vi "DUT On Logic.vi"(0 "Boolean in":refnum<vi>, 1 "reference in":refnum<vi>, 2 "Mfg. Date:":timestamp=timestamp(3431055600 s since 1904-01-01) format="%<%m/%d/%Y>T", 7 "reference 3":refnum<vi>, 9 "DeviceParameters":T1 {"DevInfo"."ASICtrim" format="%02x"}, 12 "reference 4":refnum<vi>, 13 "State-machine Local Variables in":T3={"Message"="", "Homed?"=FALSE, "NextState"=enum."Timeout", "G.Load"=1.0, "G.Position"=0.0, "Load#"=0, "[G.Loads]"=[], "[TotalLoads]"=[], "[Errors]"=[], "ZeroWait"=0, "Results"=[], "DwellWait"=FALSE, "Test Result"=FALSE, "[CondyleLoads]"=[], "[Max]"=[], "[Min]"=[], "Valid String?"=FALSE, "ScanTime"=timestamp(0 s since 1904-01-01), "ScannedString"="", "LabelDevID"=0, "MfgDate"=timestamp(0 s since 1904-01-01), "[EEPROM Cmds]"=[], "[CalData]"=[], "[A/Ds]"=[], "[A/Dmax]"=[], "[A/Dmin]"=[], "BattMax"=0.0, "BattMin"=0.0, "DwellTime"=0, "PendingDeviceType"="", "Zero G.load"=0.0, "GAINC Value"="", "Programming Step"=enum."Load EEPROM", "Front Panel Program?"=FALSE, "Final Program?"=FALSE, "PCB Score"=100, "AssyScore"=100, "Pass/Fail #"="", "Result String"="", "Programming Mode"=enum."Initial Program", "Angle Test Step"=enum."Get Y", "Accel Values"=[], "Shutdown Counter"=0, "V1"=0, "V2"=5, "V3"=0, "V4"=0, "EEPROM Data"=[], "Counter"=0, "Page#"=0, "Timer"=timestamp(0 s since 1904-01-01), "Use Mark10?"=FALSE, "Eng-Result#"=0, "DUT Serial #"=0, "Scroll Message?"=FALSE, "Clear Message"=FALSE, "Batt Test Step "=enum."Initialize", "RXTX Window Found?"=FALSE, "Shutdown First Call?"=FALSE, "A2 Delay (msec)"=0, "Support Script"={"Script #"="", "Script Revision"="", "[OEMs]"=[], "[[DeviceTypes]]"=[], "[[DeviceTypesVals]]"=[], "[[List of Errors]]"=[], "Default GAINC"="", "[[ASICtrims]]"=[], "ID For Echo"="", "Condyle A CalFactor"=100, "Condyle B CalFactor"=100, "[OEMs Prefix]"=[], "Packet ID 18"="", "[[Force Table Load Test]]"=[], "[[Force Table AccurTest]]"=[]}, "Serial Table"={"Serial File Path"=path "", "[[Serial Lookup Table]]"=[], "Serial Device Info"=[], "Valid Serial?"=FALSE}, "Target Information"={"Target Brand"="", "Target DeviceType"="", "Target Serial#"=100, "Target Lot#"=0, "Target DevID"=0, "Target Channel"=5}, "Operator"="", "COM Port"="", "Config Path"=path "", "Tx Array"=[], "DUT Parameters"={"Channel"=0, "DeviceID"=0, "Script Rev"=0, "Month"=0, "Day"=0, "Year"=0, "Lot#"=0, "V1"=0, "V2"=0, "V3"=0, "V4"=0, "MFG"=0, "Cal FactorA"=0, "Cal FactorB"=0, "ASICtrim"=[], "TmpChan"=0, "GAINC"="", "Brand"="", "Device"="", "Serial #"=0, "Batt310"=0, "Batt 280"=0}, "FTS Main?"=FALSE, "Loading"={"[Forces]"=[], "[Dwell]"=[], "Loading Step"=enum."Initialize Test"}, "Software Version"="", "Correction Factor"="", "Second Load Test"=FALSE, "Acc Loads"=[], "Mark10 Config"={"H2S%"=[80.0, 85.0, 90.0, 95.0, 100.0], "H2S Speed"=[12.0, 8.0, 6.0, 4.0, 2.0], "H to S"=2.0, "Home Speed"=1.0, "LoadWin"=0.0, "Load Speed"=0.0, "PID"={"Kp"=0.04, "Kd"=0.005001, "Ki"=2.9999999999999923e-05}}, "Channels"={"Transceiver Ch"=5, "Operating Ch"=5, "Start Ch"=0}} {"Mark10 Config"."PID"."Ki" min=0.0 max=200.0 format="%.6f"; "Mark10 Config"."PID"."Kd" min=0.0 max=200.0 format="%.6f"; "Mark10 Config"."PID"."Kp" min=0.0 max=200.0 format="%.6f"; "DUT Parameters"."ASICtrim" format="%02x"}, 14 "New Data":bool) -> (4 "Main Data out":T3={"Message"="", "Homed?"=FALSE, "NextState"=enum."Timeout", "G.Load"=1.0, "G.Position"=0.0, "Load#"=0, "[G.Loads]"=[], "[TotalLoads]"=[], "[Errors]"=[], "ZeroWait"=0, "Results"=[], "DwellWait"=FALSE, "Test Result"=FALSE, "[CondyleLoads]"=[], "[Max]"=[], "[Min]"=[], "Valid String?"=FALSE, "ScanTime"=timestamp(0 s since 1904-01-01), "ScannedString"="", "LabelDevID"=0, "MfgDate"=timestamp(0 s since 1904-01-01), "[EEPROM Cmds]"=[], "[CalData]"=[], "[A/Ds]"=[], "[A/Dmax]"=[], "[A/Dmin]"=[], "BattMax"=0.0, "BattMin"=0.0, "DwellTime"=0, "PendingDeviceType"="", "Zero G.load"=0.0, "GAINC Value"="", "Programming Step"=enum."Load EEPROM", "Front Panel Program?"=FALSE, "Final Program?"=FALSE, "PCB Score"=100, "AssyScore"=100, "Pass/Fail #"="", "Result String"="", "Programming Mode"=enum."Initial Program", "Angle Test Step"=enum."Get Y", "Accel Values"=[], "Shutdown Counter"=0, "V1"=0, "V2"=5, "V3"=0, "V4"=0, "EEPROM Data"=[], "Counter"=0, "Page#"=0, "Timer"=timestamp(0 s since 1904-01-01), "Use Mark10?"=FALSE, "Eng-Result#"=0, "DUT Serial #"=0, "Scroll Message?"=FALSE, "Clear Message"=FALSE, "Batt Test Step "=enum."Initialize", "RXTX Window Found?"=FALSE, "Shutdown First Call?"=FALSE, "A2 Delay (msec)"=0, "Support Script"={"Script #"="", "Script Revision"="", "[OEMs]"=[], "[[DeviceTypes]]"=[], "[[DeviceTypesVals]]"=[], "[[List of Errors]]"=[], "Default GAINC"="", "[[ASICtrims]]"=[], "ID For Echo"="", "Condyle A CalFactor"=100, "Condyle B CalFactor"=100, "[OEMs Prefix]"=[], "Packet ID 18"="", "[[Force Table Load Test]]"=[], "[[Force Table AccurTest]]"=[]}, "Serial Table"={"Serial File Path"=path "", "[[Serial Lookup Table]]"=[], "Serial Device Info"=[], "Valid Serial?"=FALSE}, "Target Information"={"Target Brand"="", "Target DeviceType"="", "Target Serial#"=100, "Target Lot#"=0, "Target DevID"=0, "Target Channel"=5}, "Operator"="", "COM Port"="", "Config Path"=path "", "Tx Array"=[], "DUT Parameters"={"Channel"=0, "DeviceID"=0, "Script Rev"=0, "Month"=0, "Day"=0, "Year"=0, "Lot#"=0, "V1"=0, "V2"=0, "V3"=0, "V4"=0, "MFG"=0, "Cal FactorA"=0, "Cal FactorB"=0, "ASICtrim"=[], "TmpChan"=0, "GAINC"="", "Brand"="", "Device"="", "Serial #"=0, "Batt310"=0, "Batt 280"=0}, "FTS Main?"=FALSE, "Loading"={"[Forces]"=[], "[Dwell]"=[], "Loading Step"=enum."Initialize Test"}, "Software Version"="", "Correction Factor"="", "Second Load Test"=FALSE, "Acc Loads"=[], "Mark10 Config"={"H2S%"=[80.0, 85.0, 90.0, 95.0, 100.0], "H2S Speed"=[12.0, 8.0, 6.0, 4.0, 2.0], "H to S"=2.0, "Home Speed"=1.0, "LoadWin"=0.0, "Load Speed"=0.0, "PID"={"Kp"=0.04, "Kd"=0.005001, "Ki"=2.9999999999999923e-05}}, "Channels"={"Transceiver Ch"=5, "Operating Ch"=5, "Start Ch"=0}} {"Mark10 Config"."PID"."Ki" min=0.0 max=200.0 format="%.6f"; "Mark10 Config"."PID"."Kd" min=0.0 max=200.0 format="%.6f"; "Mark10 Config"."PID"."Kp" min=0.0 max=200.0 format="%.6f"; "DUT Parameters"."ASICtrim" format="%02x"})   [LabVIEW 2013]
uses:
  Controls/Gen2 FT Globals.vi
  Controls/Gen2 FT states.ctl
  Controls/Iniial Device Programming.ctl
  ProgramStageControl.ctl
  Controls/LocalVars.ctl
  Controls/InfoPacket.ctl
  Controls/DeviceInfo.ctl
  Controls/Batt Cap Steps.ctl
  Controls/Support Script.ctl
  Controls/Serial Table.ctl
  Controls/Device Information.ctl
  Controls/Load Step.ctl
  Controls/Loading.ctl
  Controls/PID parameters.ctl
  Controls/Mark10 Config.ctl
  Controls/Channels.ctl
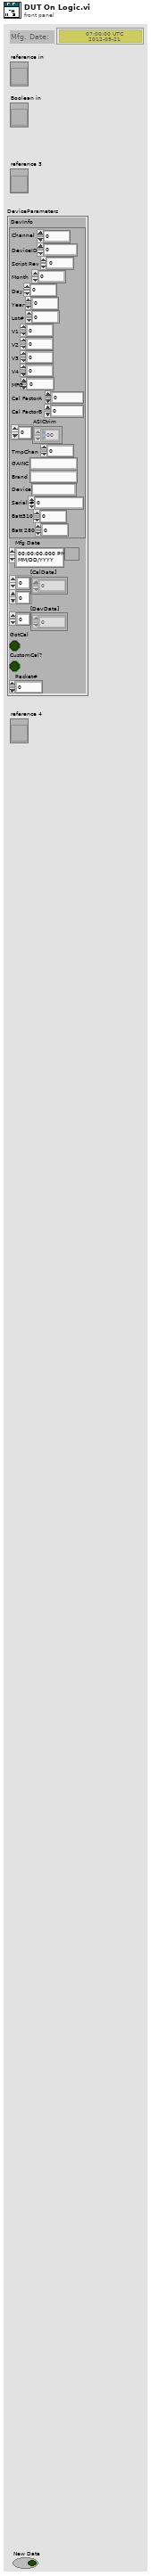
[diagram p1: front panel]
types:
  T1 = typedef "DeviceInfo.ctl" = cluster{"DevInfo":T2, "Mfg Date":timestamp, "[CalData]":u8[][], "[DevData]":u8[], "GotCal":bool, "CustomCal?":bool, "Packet#":i32}
  T2 = typedef "InfoPacket.ctl" = cluster{"Channel":u8, "DeviceID":u32, "Script Rev":u8, "Month":u8, "Day":u8, "Year":u8, "Lot#":u32, "V1":u16, "V2":u16, "V3":u16, "V4":u16, "MFG":u8, "Cal FactorA":u8, "Cal FactorB":u8, "ASICtrim":u8[], "TmpChan":u8, "GAINC":string, "Brand":string, "Device":string, "Serial #":u64, "Batt310":u16, "Batt 280":u16}
  T3 = typedef "LocalVars.ctl" = cluster{"Message":string, "Homed?":bool, "NextState":T4, "G.Load":dbl, "G.Position":dbl, "Load#":i32, "[G.Loads]":dbl[], "[TotalLoads]":dbl[], "[Errors]":dbl[][], "ZeroWait":u32, "Results":dbl[], "DwellWait":bool, "Test Result":bool, "[CondyleLoads]":dbl[][], "[Max]":dbl[], "[Min]":dbl[], "Valid String?":bool, "ScanTime":timestamp, "ScannedString":string, "LabelDevID":u32, "MfgDate":timestamp, "[EEPROM Cmds]":u8[][], "[CalData]":u8[][], "[A/Ds]":dbl[][], "[A/Dmax]":dbl[], "[A/Dmin]":dbl[], "BattMax":dbl, "BattMin":dbl, "DwellTime":i32, "PendingDeviceType":string, "Zero G.load":dbl, "GAINC Value":string, "Programming Step":T5, "Front Panel Program?":bool, "Final Program?":bool, "PCB Score":i32, "AssyScore":i32, "Pass/Fail #":string, "Result String":string, "Programming Mode":T6, "Angle Test Step":enum16{"Initialize", "Get X", "Get Y", "Get Z", "Next Test"}, "Accel Values":dbl[][], "Shutdown Counter":u32, "V1":i32, "V2":i32, "V3":i32, "V4":i32, "EEPROM Data":i32[][], "Counter":i32, "Page#":i32, "Timer":timestamp, "Use Mark10?":bool, "Eng-Result#":u32, "DUT Serial #":i32, "Scroll Message?":bool, "Clear Message":bool, "Batt Test Step ":T7, "RXTX Window Found?":bool, "Shutdown First Call?":bool, "A2 Delay (msec)":i16, "Support Script":T8, "Serial Table":T9, "Target Information":T10, "Operator":string, "COM Port":string, "Config Path":path, "Tx Array":u8[], "DUT Parameters":T2, "FTS Main?":bool, "Loading":T11, "Software Version":string, "Correction Factor":string, "Second Load Test":bool, "Acc Loads":dbl[][], "Mark10 Config":T13, "Channels":T15}
  T4 = typedef "Gen2 FT states.ctl" = enum16{"---------SETUP-------", "Initialization", "Read Support Data", "Initialize Mark-10", "Initialize Transceiver", "------UTILITIES------", "Change DUT Channel", "Find RxTx Window", "Reset Device", "Scan Channels", "Read Serial Lookup", "Shutdown Device", "ESTOP", "--------USER---------", "Timeout", "-----PROGRAM-----", "Program Device", "------MARK10--------", "Go Home", "MoveUp", "MoveDown", "Goto Load", "Goto Position", "Stop Motor", "---------TESTS--------", "Start Test", "Angle Test", "Load Test", "Load Accuracy Test", "Battery Test", "------RESULTS-------", "End Test", "Display Result", "--------EXIT--------", "Exit"}
  T5 = typedef "Iniial Device Programming.ctl" = enum16{"Load EEPROM", "Send First A1", "Send EEPROM", "Send A1", "Check EEPROM Echo", "Verify transmission", "Programming Successful", "Programming Failed"}
  T6 = typedef "ProgramStageControl.ctl" = enum16{"Initial Program", "GainC", "Scales"}
  T7 = typedef "Batt Cap Steps.ctl" = enum16{"Initialize", "Collect 2.8 Volts", "Collect 3.1 Volts", "Check Results"}
  T8 = typedef "Support Script.ctl" = cluster{"Script #":string, "Script Revision":string, "[OEMs]":string[], "[[DeviceTypes]]":string[][], "[[DeviceTypesVals]]":u16[][], "[[List of Errors]]":string[][], "Default GAINC":string, "[[ASICtrims]]":u8[][], "ID For Echo":string, "Condyle A CalFactor":i32, "Condyle B CalFactor":i32, "[OEMs Prefix]":string[], "Packet ID 18":string, "[[Force Table Load Test]]":dbl[][], "[[Force Table AccurTest]]":dbl[][]}
  T9 = typedef "Serial Table.ctl" = cluster{"Serial File Path":path, "[[Serial Lookup Table]]":string[][], "Serial Device Info":string[], "Valid Serial?":bool}
  T10 = typedef "Device Information.ctl" = cluster{"Target Brand":string, "Target DeviceType":string, "Target Serial#":i32, "Target Lot#":u32, "Target DevID":u32, "Target Channel":u8}
  T11 = typedef "Loading.ctl" = cluster{"[Forces]":dbl[], "[Dwell]":dbl[], "Loading Step":T12}
  T12 = typedef "Load Step.ctl" = enum16{"Initialize Test", "Go Home", "Detect Dev Surface", "Wait to zero Device", "Zero Device", "Do Test", "Test Result"}
  T13 = typedef "Mark10 Config.ctl" = cluster{"H2S%":dbl[], "H2S Speed":dbl[], "H to S":dbl, "Home Speed":dbl, "LoadWin":dbl, "Load Speed":dbl, "PID":T14}
  T14 = typedef "PID parameters.ctl" = cluster{"Kp":dbl, "Kd":dbl, "Ki":dbl}
  T15 = typedef "Channels.ctl" = cluster{"Transceiver Ch":u8, "Operating Ch":u8, "Start Ch":u8}
  T16 = typedef "LVDateTimeRec.ctl" = cluster{"fractional second":dbl, "second":i32, "minute":i32, "hour":i32, "day of month":i32, "month":i32, "year":i32, "day of week":i32, "day of year":i32, "DST":i32}
  T17 = typedef "InfoPacket.ctl" = cluster{"Channel":u8, "DeviceID":u32, "Script Rev":u8, "Month":u8, "Day":u8, "Year":u8, "Lot#":u32, "V1":u16, "V2":u16, "V3":u16, "V4":u16, "MFG":u8, "Cal Factor":u8, "Cal FactorB":u8, "ASICtrim":u8[], "TmpChan":u8, "GAINC Value":string, "Brand":string, "DeviceType":string, "Serial Number":u64}
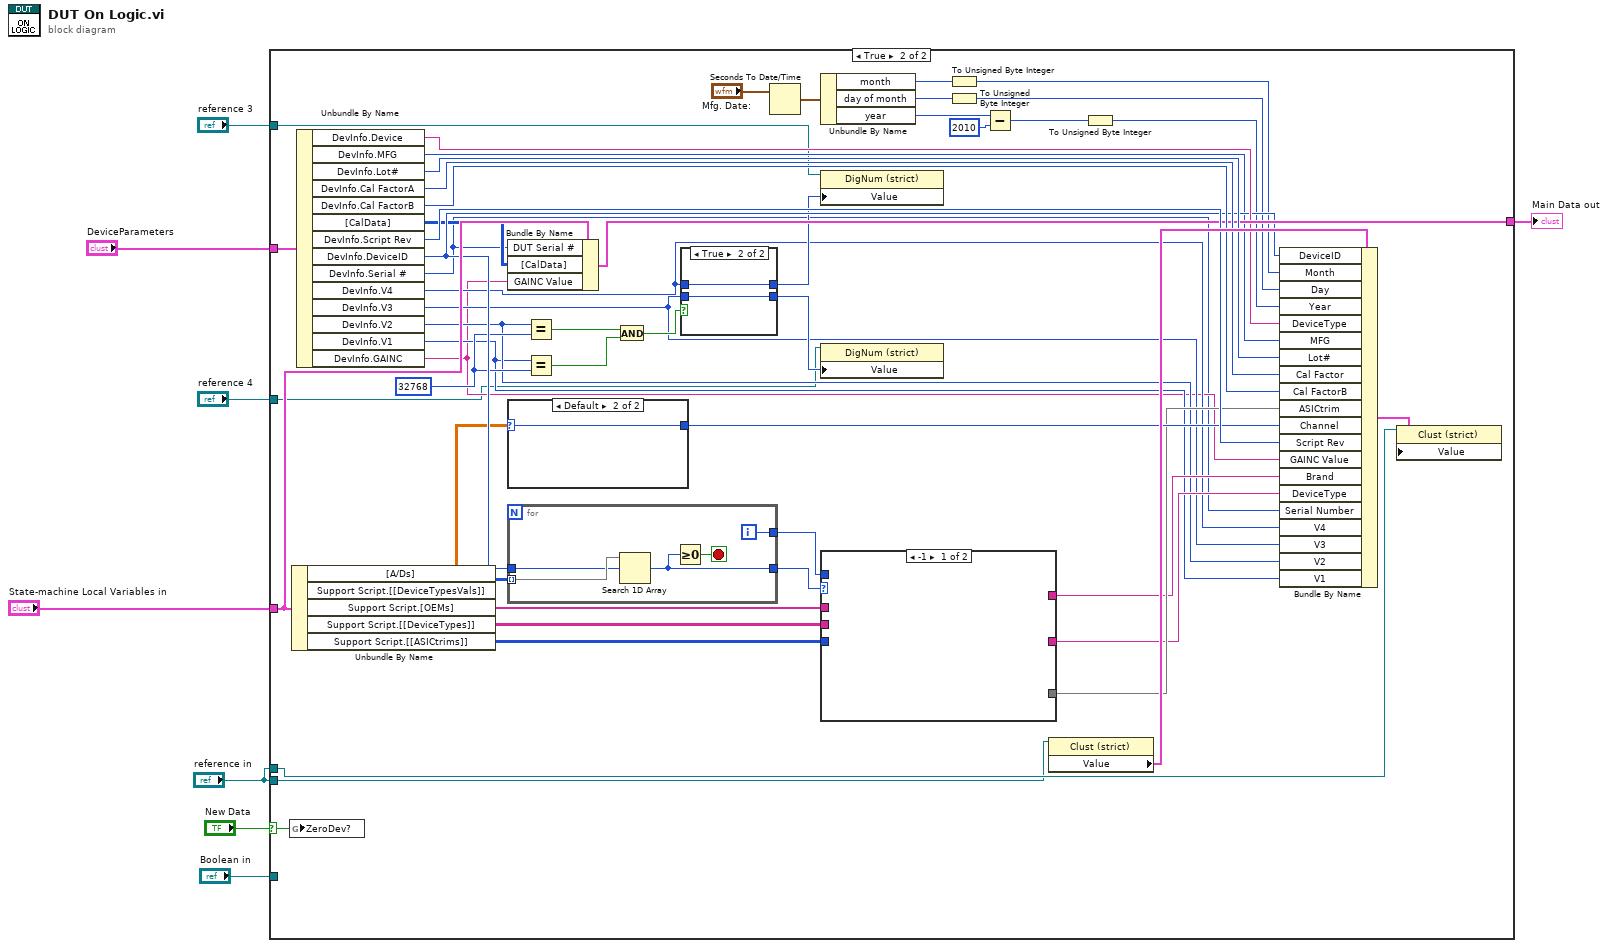
[diagram p0: block diagram]
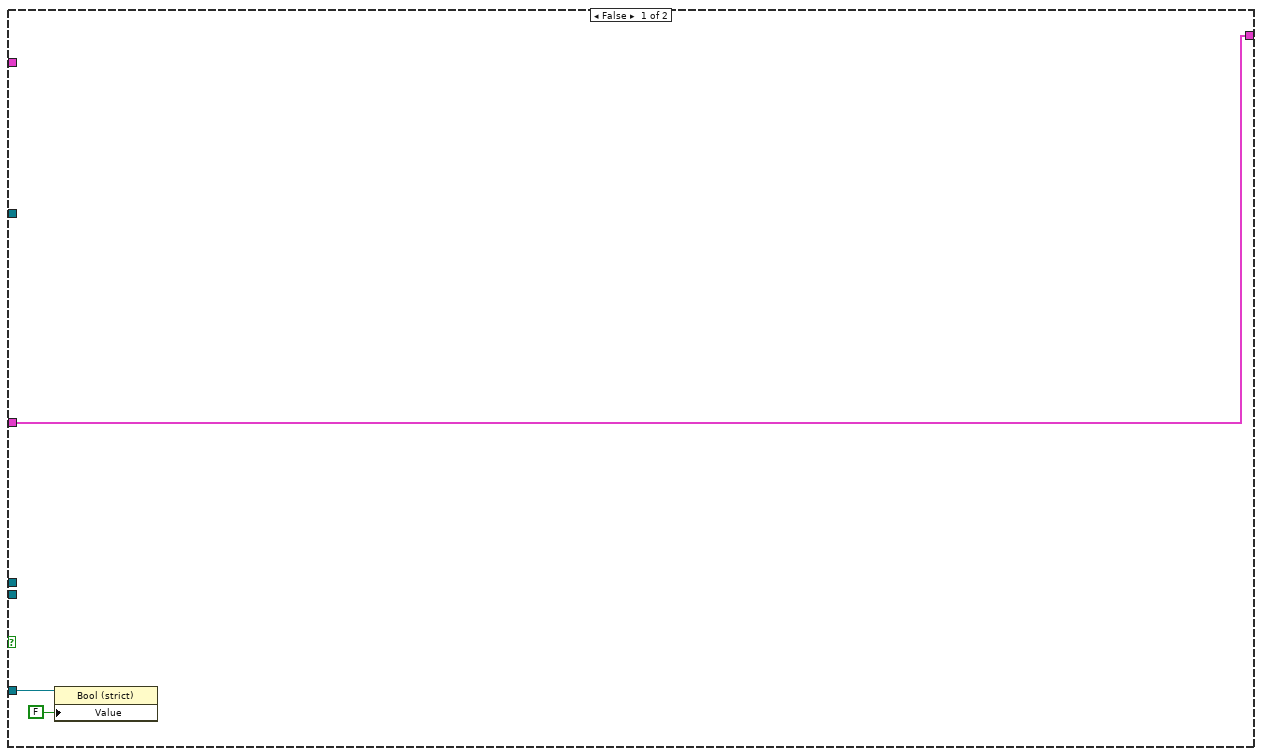
[diagram p2: hidden frame]
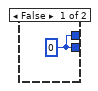
[diagram p3: hidden frame]
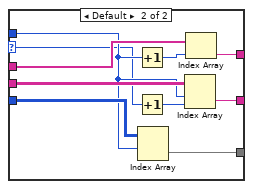
[diagram p4: hidden frame]
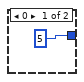
[diagram p5: hidden frame]
diagram:
  n1 = case shown="True" "New Data" {
    selector: "New Data" -> [_ w30]
    tunnel: "DeviceParameters" -> [_ w60]
    tunnel: [w11 w48] -> w6
    tunnel: "State-machine Local Variables in" -> [w11 w47]
    tunnel: "Boolean in" -> [w9 _]
    tunnel: "reference in" -> [_ w17]
    tunnel: "reference in" -> [_ w16]
    tunnel: "reference 3" -> [_ w15]
    tunnel: "reference 4" -> [_ w14]
    frame False {
      n2 = property class="Bool (strict)"(reference=w9, "Value"=FALSE ("Device ON?")) -> ()  [unwired: 1 in, 2 out]
    }
    frame True {
      w29 = 32768
      n3 = global write "Gen2 FT Globals.vi" "ZeroDev?"(w30) -> ()
      n4 = Unbundle By Name(w47) -> ("[A/Ds]"=w13:dbl[][], "Support Script.[[DeviceTypesVals]]"=w46:u16[][], "Support Script.[OEMs]"=w41:string[], "Support Script.[[DeviceTypes]]"=w42:string[][], "Support Script.[[ASICtrims]]"=w45:u8[][])
      n5 = Unbundle By Name(w60) -> ("DevInfo.Device"=w40:string, "DevInfo.MFG"=w18:u8, "DevInfo.Lot#"=w52:u32, "DevInfo.Cal FactorA"=w59:u8, "DevInfo.Cal FactorB"=w51:u8, "[CalData]"=w35:u8[][], "DevInfo.Script Rev"=w50:u8, "DevInfo.DeviceID"=w36:u32, "DevInfo.Serial #"=w12:u64, "DevInfo.V4"=w20:u16, "DevInfo.V3"=w22:u16, "DevInfo.V2"=w28:u16, "DevInfo.V1"=w27:u16, "DevInfo.GAINC"=w19:string)
      n6 = Bundle By Name(cluster=w47, "DUT Serial #"=w12, "[CalData]"=w35, "GAINC Value"=w19) -> (w48:T3)
      n7 = case shown="Default" w13 {
        selector: w13 -> [_ w82]
        tunnel: [u8 5 ("RF Channel:") w82] -> w49
        frame 0 {
        }
        frame Default {
        }
      }
      n8 = for {
        tunnel: w46 -> [w80] mode=indexing
        tunnel: [w78] -> w39
        tunnel: w36 -> [w77]
        tunnel: [w76] -> w43
        i -> [w76]
        stop <- w79 stop-if-true
        n9 = Search 1D Array(1D array=w80, element=w77) -> (index of element=w78:i32)  [unwired: 1 in]
        n10 = Greater Or Equal To 0?(x=w78) -> (x >= 0?=w79:bool)
      }
      n11 = Equal?(x=w28, y=w29) -> (x = y?=w26:bool)
      n12 = Equal?(x=w27, y=w29) -> (x = y?=w25:bool)
      n13 = And(x=w26, y=w25) -> (x .and. y?=w24:bool)
      n14 = case shown="True" w24 {
        tunnel: [w63 w65] -> w23
        tunnel: w22 -> [_ w65]
        tunnel: [w63 w64] -> w21
        tunnel: w20 -> [_ w64]
        frame False {
          w63 = 0
        }
        frame True {
        }
      }
      n15 = Seconds To Date/Time(time stamp (now)="Mfg. Date:") -> (date time rec=w57:T16)  [unwired: 1 in]
      n16 = Unbundle By Name(w57) -> ("month"=w56:i32, "day of month"=w55:i32, "year"=w54:i32)
      n17 = property class="DigNum (strict)"(reference=w15, "Value"=w21) -> ()  [unwired: 1 in, 2 out]
      n18 = property class="DigNum (strict)"(reference=w14, "Value"=w23) -> ()  [unwired: 1 in, 2 out]
      n19 = case shown="-1" w39 {
        selector: w39 -> [_ w66]
        tunnel: w42 -> [_ w75]
        tunnel: w41 -> [_ w74]
        tunnel: w43 -> [_ w69]
        tunnel: [_ w73] -> w37
        tunnel: [_ w72] -> w38
        tunnel: w45 -> [_ w70]
        tunnel: [_ w68] -> w44
        frame -1 {
        }
        frame Default {
          n20 = Increment(x=w69) -> (x+1=w71:i32)
          n21 = Increment(x=w66) -> (x+1=w67:i32)
          n22 = Index Array(array=w70, index (row)=w69) -> (element=w68:u8[])  [unwired: 1 in]
          n23 = Index Array(array=w75, index (row)=w69, index (col)=w67) -> (element=w73:string)
          n24 = Index Array(array=w74, index=w71) -> (element=w72:string)
        }
      }
      n25 = To Unsigned Byte Integer(number=w56) -> (unsigned 8bit integer=w33:u8)
      n26 = To Unsigned Byte Integer(number=w55) -> (unsigned 8bit integer=w32:u8)
      n27 = Subtract(x=w54, y=2010) -> (x-y=w58:i32)
      n28 = property class="Clust (strict)"(reference=w16) -> ("Value"=w61:T17)  [unwired: 1 in, 2 out]
      n29 = To Unsigned Byte Integer(number=w58) -> (unsigned 8bit integer=w31:u8)
      n30 = Bundle By Name(cluster=w61, "DeviceID"=w36, "Month"=w33, "Day"=w32, "Year"=w31, "DeviceType"=w40, "MFG"=w18, "Lot#"=w52, "Cal Factor"=w59, "Cal FactorB"=w51, "ASICtrim"=w44, "Channel"=w49, "Script Rev"=w50, "GAINC Value"=w19, "Brand"=w38, "DeviceType"=w37, "Serial Number"=w12, "V4"=w20, "V3"=w22, "V2"=w28, "V1"=w27) -> (w62:T17)
      n31 = property class="Clust (strict)"(reference=w17, "Value"=w62) -> ()  [unwired: 1 in, 2 out]
    }
  }
  "Main Data out" <- w6
